vi "ReadTraces.vi"(8 "error in (no error)":errorcluster) -> (0 "error out":errorcluster, 2 "All elements":cluster{string[]}[](array[cluster]))   [LabVIEW 2018]
uses:
  protected/Tracer_ClassAttributes.vi
  Tracer.lvclass
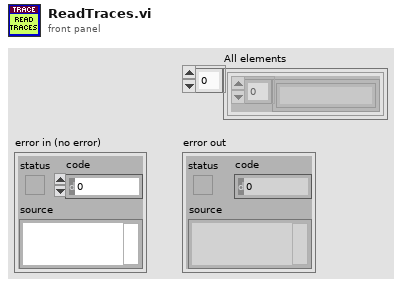
[diagram p1: front panel]
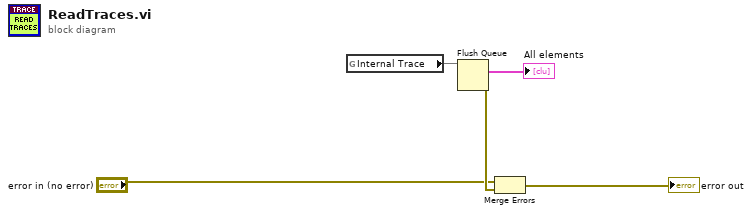
[diagram p0: block diagram]
diagram:
  n1 = global read "Tracer_ClassAttributes.vi" "Internal Trace"() -> (w1)
  n2 = Flush Queue(queue=w1) -> (remaining elements=→"All elements":cluster{string[]}[], error out=w5:errorcluster)  [unwired: 1 in, 1 out]
  n3 = Merge Errors("error in (no error)", w5) -> (→"error out":errorcluster)
